vi "User Interface.vi"() -> ()   [LabVIEW 2017, in "DSF Core.lvlib"]
uses:
  DSF Core.lvlib
  Components/Transceivers/UDP/UI/UDP UI.lvclass
  C:/Git/DSF/Core/Classes/Component User Interface/Component User Interface.lvclass
  Typedefs/DSF Version Info.ctl
  Components/Transceivers/UDP/Configuration/UDP Configuration.lvclass
  C:/Git/DSF/Core/Classes/Component Configuration/Component Configuration.lvclass
  Classes/User Interface/User Interface.lvclass
  Classes/Component User Interface/Component User Interface.lvclass
  Classes/Configuration/Configuration.lvclass
  Classes/User Interface Events/User Interface Events.lvclass
panel:
  out "json":string="{\"local port\":0,\"local address\":0}"
  in  "stop":bool
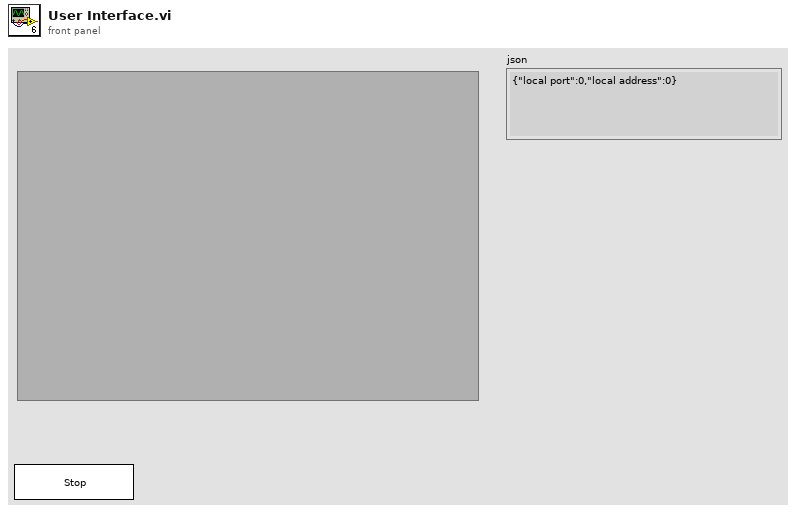
[diagram p1: front panel]
types:
  T1 = typedef "DSF Core.lvlib/DSF Version Info.ctl" = cluster{"major":u32, "minor":u32, "fix":u32, "build":string}
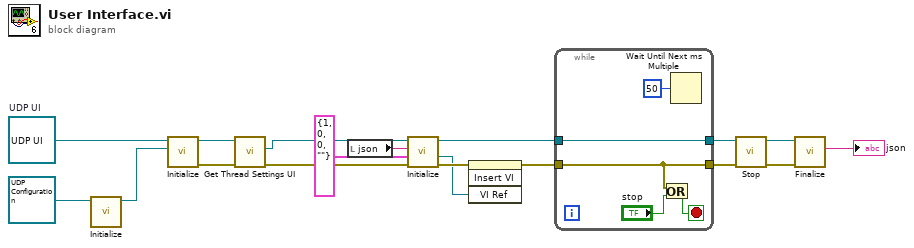
[diagram p0: block diagram]
diagram:
  w17 = refnum<class "UDP UI.lvclass"> refnum  # UDP UI
  n1 = call-dynamic "Initialize.vi"("UDP Configuration in"=refnum<class "UDP Configuration.lvclass"> refnum ("DSF Core.lvlib:UDP Configuration.lvclass")) -> ("UDP Configuration out"=w13:refnum<class "UDP Configuration.lvclass">)  [unwired: 9 in, 1 out]
  n2 = call-dynamic "Initialize.vi"("Component Configuration"=w13, "UDP UI in"=w17) -> ("error out"=w15:errorcluster, "UDP UI out"=w16:refnum<class "UDP UI.lvclass">)  [unwired: 8 in]
  n3 = call "Get Thread Settings UI.vi"("error in (no error)"=w15, "Component UI in"=w16) -> ("error out"=w12:errorcluster, "Thread Settings UI"=w11:refnum<class "User Interface.lvclass">)  [unwired: 7 in, 1 out]
  n4 = local read "json"() -> (w9:string)
  n5 = call-dynamic "Initialize.vi"("error in (no error)"=w12, "json version"=T1 {"major"=1, "minor"=0, "fix"=0, "build"=""} ("version"), "json"=w9, "User Interface in"=w11) -> ("error out"=w8:errorcluster, "vi ref"=w7:refnum<vi>, "User Interface out"=w6:refnum<class "User Interface.lvclass">)  [unwired: 4 in, 1 out]
  n6 = invoke on="Sub Panel" class="SubPnl" method="Insert VI"(error in=w8, "VI Ref"=w7) -> (error out=w18:errorcluster)  [unwired: 2 in, 3 out]
  n7 = while {
    tunnel: w18 -> [w22]
    tunnel: [w22] -> w4
    tunnel: w6 -> [w19]
    tunnel: [w19] -> w5
    stop <- w20 stop-if-true
    n8 = Or(x=w22, y="stop") -> (x .or. y?=w20:bool)
    n9 = Wait Until Next ms Multiple(millisecond multiple=u32 50) -> ()  [unwired: 1 out]
  }
  n10 = call "Stop.vi"("error in (no error)"=w4, "User Interface in"=w5) -> ("error out"=w2:errorcluster, "User Interface out"=w3:refnum<class "User Interface.lvclass">)  [unwired: 8 in]
  n11 = call-dynamic "Finalize.vi"("error in (no error)"=w2, "User Interface in"=w3) -> ("json"=→"json":string)  [unwired: 6 in, 3 out]
